vi "RS-232C_USB.vi"() -> ()   [LabVIEW 2017]
uses:
  <vilib>/Instr/_visa.llb/VISA Configure Serial Port (Instr).vi
panel:
  in  "タイムアウト":u32=10
  in  "速度":string(combo)="9600"
  out "受信文字列":string
  in  "終了ボタン":bool
  in  "送信ボタン":bool
  in  "クリアボタン":bool
  in  "VISA resource name":refnum<visa-resource-name> caption="COMポート"
  in  "コマンド":string="*IDN?"
  # "秒"
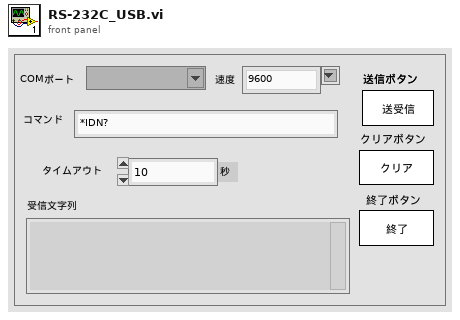
[diagram p1: front panel]
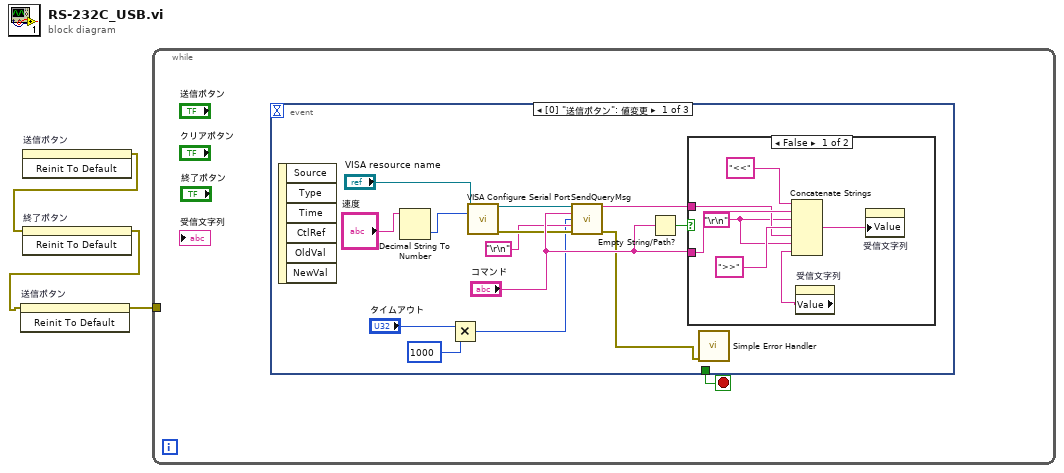
[diagram p0: block diagram]
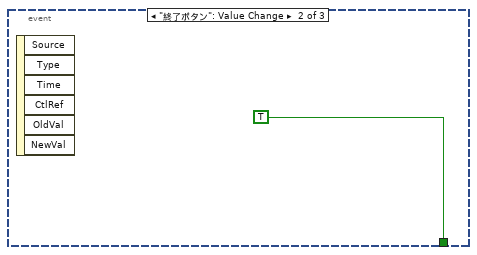
[diagram p3: hidden frame]
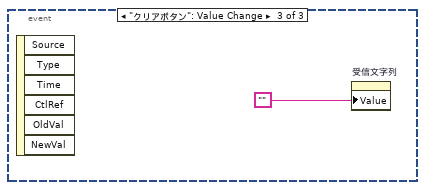
[diagram p4: hidden frame]
diagram:
  n1 = invoke on="送信ボタン" class="Bool" method="Reinit To Default"() -> (error out=w3:errorcluster)  [unwired: 3 in, 2 out]
  n2 = invoke on="終了ボタン" class="Bool" method="Reinit To Default"(error in=w3) -> (error out=w2:errorcluster)  [unwired: 2 in, 2 out]
  n3 = invoke on="送信ボタン" class="Bool" method="Reinit To Default"(error in=w2) -> (error out=w1:errorcluster)  [unwired: 2 in, 2 out]
  n4 = while {
    tunnel: w1 -> [_]
    stop <- w4 stop-if-true
    n5 = event shown="[0] \"送信ボタン\": 値変更" {
      selector: _ -> [_ _ _]
      dyn-events: _ -> [_ _ _]
      timeout: _ -> [_ _ _]
      tunnel: [_ TRUE _] -> w4
      event "送信ボタン": Value Change {
        n6 = event-data() -> ()  [unwired: 1 in, 6 out]
        n7 = Decimal String To Number(string="速度") -> (number=w15:i32)  [unwired: 2 in, 1 out]
        n8 = Multiply(x="タイムアウト", y=u32 1000) -> (x*y=w5:u32)
        n9 = call-poly "VISA Configure Serial Port"("VISA resource name"="VISA resource name", "baud rate (9600)"=w15) -> ("VISA resource name out"=w13:refnum<visa-resource-name>, "error out"=w11:errorcluster)  [unwired: 12 in]
        n10 = call "SendQueryMsg.vi"("VISAリソース名"=w13, "入力文字列"="コマンド", "タイムアウト"=w5, "ターミネータ"="\r\n", "エラー入力"=w11) -> ("受信文字列"=w9:string, "エラー出力"=w10:errorcluster)  [unwired: 9 in]
        n11 = Empty String/Path?(string/path="コマンド") -> (empty?=w14:bool)
        n12 = case shown="FALSE" w14 {
          tunnel: "コマンド" -> [w24 _]
          tunnel: w9 -> [w21 _]
          frame False {
            w18 = "\r\n"
            n13 = property on="受信文字列" class="Str"() -> ("Value"=w19:string)  [unwired: 2 in, 2 out]
            n14 = Concatenate Strings("<<", w24, w18, ">>", w21, w18, w19) -> (w20:string)
            n15 = property on="受信文字列" class="Str"("Value"=w20) -> ()  [unwired: 2 in, 2 out]
          }
          frame True {
          }
        }
        n16 = call <vilib>:"Simple Error Handler.vi"("error in (no error)"=w10) -> ()  [unwired: 4 in, 5 out]
      }
      event "終了ボタン": Value Change {
        n17 = event-data() -> ()  [unwired: 1 in, 6 out]
      }
      event "クリアボタン": Value Change {
        n18 = event-data() -> ()  [unwired: 1 in, 6 out]
        n19 = property on="受信文字列" class="Str"("Value"="") -> ()  [unwired: 2 in, 2 out]
      }
    }
  }
